vi "Switchmatrix Loop.vi"(6 "Used functions":bool, 8 "error in":errorcluster, 9 "IBM OptoElectroMechanics Configuration":T1={"Parameter Analizer"={"Parameter Analyzer VISA Session"="COM1", "Sweeping Time Parameters"={"Integration Time"=0, "Short Integration Time (s)"=1.0, "Long Integration Time (s)"=0.0, "Wait Time Parameter"=1.0}, "Acquisition Mode"=enum."Sweeping Mode", "Status Polling Time (ms)"=0, "Comment"="Test VI", "SMU 1 - Sweeping"={"Start / Offset"=0.0, "Stop / Ratio"=1.0, "Step \n(linear only)"=0.01, "Compliance"=0.1, "Power \nCompliance"=0.0, "Mode"=0, "Function"=0, "Sweep Mode"=FALSE}, "SMU 2 - Sweeping"={"Start / Offset"=0.0, "Stop / Ratio"=1.0, "Step \n(linear only)"=0.01, "Compliance"=0.1, "Power \nCompliance"=0.0, "Mode"=0, "Function"=0, "Sweep Mode"=FALSE}, "SMU 3 - Sweeping"={"Start / Offset"=0.0, "Stop / Ratio"=1.0, "Step \n(linear only)"=0.01, "Compliance"=0.1, "Power \nCompliance"=0.0, "Mode"=0, "Function"=0, "Sweep Mode"=FALSE}, "SMU 4 - Sweeping"={"Start / Offset"=0.0, "Stop / Ratio"=1.0, "Step \n(linear only)"=0.01, "Compliance"=0.1, "Power \nCompliance"=0.0, "Mode"=0, "Function"=0, "Sweep Mode"=FALSE}, "Sweep Spacing"=0, "Range"=0, "SMU1 - Sampling"={"Source"=10.0, "Compliance"=1e-05, "Mode"=0, "Function"=FALSE}, "SMU2 - Sampling"={"Source"=1.0, "Compliance"=1.0, "Mode"=0, "Function"=FALSE}, "SMU3 - Sampling"={"Source"=10.0, "Compliance"=1e-05, "Mode"=0, "Function"=FALSE}, "SMU4 - Sampling"={"Source"=0.1, "Compliance"=60.0, "Mode"=10, "Function"=FALSE}, "Sampling Time Parameters"={"Initial Interval (s)"=0.1, "Number of Samples"=60, "Total Sampling Time (s)"=10.0, "Hold Time (s)"=0.0, "Sampling Mode"=0, "Sampling Time"=0}, "Stop Condition"={"Enable Delay (s)"=0.0, "Name"="", "Threshold"=0.0, "num. of events"=1, "Event"=0, "Stop Condition Enable"=FALSE}}, "Switching Matrix"={"Switching Matrix VISA Session"="GPIB0::18::INSTR", "Connections"=[{"Connections"=[FALSE, FALSE, FALSE, FALSE, FALSE, FALSE, FALSE, FALSE, FALSE, FALSE, FALSE, FALSE], "Connection Type"=enum."Disconnected"}, {"Connections"=[FALSE, FALSE, FALSE, FALSE, FALSE, FALSE, FALSE, FALSE, FALSE, FALSE, FALSE, FALSE], "Connection Type"=enum."Disconnected"}, {"Connections"=[FALSE, FALSE, FALSE, FALSE, FALSE, FALSE, FALSE, FALSE, FALSE, FALSE, FALSE, FALSE], "Connection Type"=enum."Disconnected"}, {"Connections"=[FALSE, FALSE, FALSE, FALSE, FALSE, FALSE, FALSE, FALSE, FALSE, FALSE, FALSE, FALSE], "Connection Type"=enum."Disconnected"}, {"Connections"=[FALSE, FALSE, FALSE, FALSE, FALSE, FALSE, FALSE, FALSE, FALSE, FALSE, FALSE, FALSE], "Connection Type"=enum."Disconnected"}, {"Connections"=[FALSE, FALSE, FALSE, FALSE, FALSE, FALSE, FALSE, FALSE, FALSE, FALSE, FALSE, FALSE], "Connection Type"=enum."Disconnected"}, {"Connections"=[FALSE, FALSE, FALSE, FALSE, FALSE, FALSE, FALSE, FALSE, FALSE, FALSE, FALSE, FALSE], "Connection Type"=enum."Disconnected"}, {"Connections"=[FALSE, FALSE, FALSE, FALSE, FALSE, FALSE, FALSE, FALSE, FALSE, FALSE, FALSE, FALSE], "Connection Type"=enum."Disconnected"}]}, "Stress Control"={"Stress Control VISA Session"="StrainMotor", "Axis"=0, "Motion"=0, "Destination (°)"=0.0, "Speed (°/s)"=4.0, "Position (°)"=25.0}, "Optical Spectrometer"={"Laser Settings"={"Laser Wavelength"=enum."365 nm", "Neutral Density Filter"=enum."100%"}, "Spectrometer Settings"={"Confocal Hole Size (µm)"=0.0, "Grating"=2, "Detector"=enum."InGaAs Array"}, "Acquisition Settings"={"Acquisition Mode"=enum."Multi-Window", "Spectal Position (nm)"=632.0, "From (nm)"=735.0, "To (nm)"=0.0, "Integration Time (s)"=0.0, "Number of Accumulations"=3, "AutoScanning"=FALSE, "Spike Removal"=FALSE}, "Path"=path "C:/07 - Prizes and Awards/Marie Curie Prize/Reply Editors Final NCOMMS(10).docx"}, "Switches & Mirrors"={"Relay VISA Session"="COM1", "Switches"={"Laser"=FALSE, "Video"=FALSE}, "Delays (ms)"={"Laser"=500, "Video"=1500}}, "Camera"={"Settings"={"Pixel clock"=20, "Frame rate"=30.0, "Exposure time"=33.21525, "Master Gain"=0, "Red Gain"=0, "Green Gain"=0, "Blue Gain"=0, "Auto Gain"=FALSE, "White-balance"=FALSE, "Color Correction"=FALSE}}, "XYZ Stage"={"Connection Settings"={"Tango VISA"="", "Baudrate"=57600, "Show Protocol?"=FALSE}, "Manual Control"={"North"=FALSE, "South"=FALSE, "West"=FALSE, "East"=FALSE, "Up"=FALSE, "Down"=FALSE, "Stop"=FALSE, "XY Step"=0.0, "Z step"=0.0}, "Coordinate Control"={"Motion Mode"=enum."Absolute", "Destination [mm]"=[]}}, "AutoFocus"={"Matching Criteria"={"Minimum Score"=700.0, "Color Score Weight"=700.0, "Minimum Contrast"=50, "Match Mode"=0, "Match Feature Mode"=0, "Subpixel Accuracy"=TRUE, "Color Sensitivity"=1, "Search Strategy"=1}, "Z Scan Parameters"={"Z Range"=1380.0, "Resolution"=5000.0, "Initial Direction"=enum."Up", "Focus Threshold"=0.1, "Ascent Constant"=0.1}, "Displacement"=0.0, "Transformation Matrix"=[]}, "Sava Data"={"Workspace Info"={"Device Name"="ProberHead_Tst_C29K3_7(2)", "Device Info"="ProberHead_Tst_C29", "Path"=path "C:/Users/gio/Desktop/ProbeHeadTest"}, "Instrument Configuration"={"Instrument"=enum."Unknown Instrument", "Configuration"="Test Configuration"}, "Stress Motor Position"=0.0, "Electrical Measurement"={"Sequence"=[], "V1"=[], "V2"=[], "V3"=[], "V4"=[], "I1"=[], "I2"=[], "I3"=[], "I4"=[]}, "Optical Spectrum"={"Intensity"=[], "Wavelength"=[], "Energy"=[], "Raman Shift"=[], "Detector Temperature"=0.0}}, "PlotData"={"Sliders"={"Strain Sequence"=0, "Instrument Sequence"=0}, "Measurement"={"Which Instrument?"=enum."No Plot", "Electrical Measurement"={"Sequence"=[], "V1"=[], "V2"=[], "V3"=[], "V4"=[], "I1"=[], "I2"=[], "I3"=[], "I4"=[]}, "Measurement Mode"=enum."Sweeping Mode", "Optical Spectrum"={"Intensity"=[], "Wavelength"=[], "Energy"=[], "Raman Shift"=[], "Detector Temperature"=0.0}}, "Instrument Steps"=[], "Strain Points"=[]}, "Instrument Sequence"={"Caller VI"=enum."User"}, "Strain Measurement"={"Stress Sequence "={"Max Motor Position"=1380.0, "# Intermediate Points"=5000, "Initial Direction"=enum."Tension"}, "Track?"=FALSE}} {"AutoFocus"."Displacement" scale=1.0..1000.0; "AutoFocus"."Z Scan Parameters"."Focus Threshold" min=0.0 max=1000.0 step=1.0 format="%#_2f"; "AutoFocus"."Z Scan Parameters"."Ascent Constant" min=0.0 max=1000.0 step=1.0 format="%#_2f"; "AutoFocus"."Z Scan Parameters"."Resolution" min=0.0 max=1.0 step=0.01 format="%_2g"; "AutoFocus"."Z Scan Parameters"."Z Range" format="%_3g"; "AutoFocus"."Matching Criteria"."Match Mode" items=["Shift Invariant", "Rotation Invariant"]; "AutoFocus"."Matching Criteria"."Match Feature Mode" items=["Color and Shape", "Color", "Shape"]; "AutoFocus"."Matching Criteria"."Color Sensitivity" items=["Low Sensitivity", "Medium Sensitivity", "High Sensitivity"]; "AutoFocus"."Matching Criteria"."Search Strategy" items=["Conservative", "Balance", "Aggressive", "Very Aggressive"]; "XYZ Stage"."Manual Control"."Z step" scale=0.1..10.0; "XYZ Stage"."Manual Control"."XY Step" scale=0.1..1000.0; "Camera"."Settings"."Blue Gain" min=0 max=100 scale=0.0..100.0; "Camera"."Settings"."Green Gain" min=0 max=100 scale=0.0..100.0; "Camera"."Settings"."Red Gain" min=0 max=100 scale=0.0..100.0; "Camera"."Settings"."Master Gain" min=0 max=100 scale=0.0..100.0; "Camera"."Settings"."Exposure time" min=0.101625 max=159.246375 step=0.101625 scale=0.101625..159.246375 scale format="%#.3g"; "Camera"."Settings"."Frame rate" min=2.7455631699174137 max=6.2675785993528725 step=0.000101625 scale=2.7455631699174137..6.2675785993528725 scale format="%^#_3g"; "Camera"."Settings"."Pixel clock" min=5 max=43 scale=5.0..43.0; "PlotData"."Sliders"."Instrument Sequence" scale=0.0..10.0; "PlotData"."Sliders"."Strain Sequence" scale=0.0..10.0; "Strain Measurement"."Stress Sequence"."# Intermediate Points" max=1390; "Parameter Analizer"."Stop Condition"."Event" items=["Value > Threshold", "Value < Threshold", "| Value | > | Threshold |", "| Value | < | Threshold |"]; "Parameter Analizer"."Stop Condition"."Threshold" format="%^.2e"; "Parameter Analizer"."Stop Condition"."Enable Delay (s)" format="%.1f"; "Parameter Analizer"."Sampling Time Parameters"."Sampling Time" items=["Auto (linear only)", "No Limit", "Set Limit"]; "Parameter Analizer"."Sampling Time Parameters"."Sampling Mode" items=["Linear", "Log10", "Log25", "Log50", "Thinned Out"]; "Parameter Analizer"."Sampling Time Parameters"."Hold Time (s)" format="%.4f"; "Parameter Analizer"."Sampling Time Parameters"."Total Sampling Time (s)" format="%.1f"; "Parameter Analizer"."Sampling Time Parameters"."Initial Interval (s)" format="%^.3e"; "Parameter Analizer"."SMU 4 - Sweeping"."Function" items=["Disabled", "Var 1", "Var 2", "Var 1'", "Constant"]; "Parameter Analizer"."SMU 4 - Sweeping"."Mode" items=["V", "I", "V pulse", "I  pulse", "Common"]; "Parameter Analizer"."SMU 4 - Sweeping"."Power \nCompliance" format="%^.2e"; "Parameter Analizer"."SMU 4 - Sweeping"."Compliance" format="%^.2e"; "Parameter Analizer"."SMU 4 - Sweeping"."Step \n(linear only)" format="%^.4e"; "Parameter Analizer"."SMU 4 - Sweeping"."Stop / Ratio" format="%^.4e"; "Parameter Analizer"."SMU 4 - Sweeping"."Start / Offset" format="%^.4e"; "Parameter Analizer"."SMU 3 - Sweeping"."Function" items=["Disabled", "Var 1", "Var 2", "Var 1'", "Constant"]; "Parameter Analizer"."SMU 3 - Sweeping"."Mode" items=["V", "I", "V pulse", "I  pulse", "Common"]; "Parameter Analizer"."SMU 3 - Sweeping"."Power \nCompliance" format="%^.2e"; "Parameter Analizer"."SMU 3 - Sweeping"."Compliance" format="%^.2e"; "Parameter Analizer"."SMU 3 - Sweeping"."Step \n(linear only)" format="%^.4e"; "Parameter Analizer"."SMU 3 - Sweeping"."Stop / Ratio" format="%^.4e"; "Parameter Analizer"."SMU 3 - Sweeping"."Start / Offset" format="%^.4e"; "Parameter Analizer"."SMU 2 - Sweeping"."Function" items=["Disabled", "Var 1", "Var 2", "Var 1'", "Constant"]; "Parameter Analizer"."SMU 2 - Sweeping"."Mode" items=["V", "I", "V pulse", "I  pulse", "Common"]; "Parameter Analizer"."SMU 2 - Sweeping"."Power \nCompliance" format="%^.2e"; "Parameter Analizer"."SMU 2 - Sweeping"."Compliance" format="%^.2e"; "Parameter Analizer"."SMU 2 - Sweeping"."Step \n(linear only)" format="%^.4e"; "Parameter Analizer"."SMU 2 - Sweeping"."Stop / Ratio" format="%^.4e"; "Parameter Analizer"."SMU 2 - Sweeping"."Start / Offset" format="%^.4e"; "Parameter Analizer"."SMU 1 - Sweeping"."Function" items=["Disabled", "Var 1", "Var 2", "Var 1'", "Constant"]; "Parameter Analizer"."SMU 1 - Sweeping"."Mode" items=["V", "I", "V pulse", "I  pulse", "Common"]; "Parameter Analizer"."SMU 1 - Sweeping"."Power \nCompliance" format="%^.2e"; "Parameter Analizer"."SMU 1 - Sweeping"."Compliance" format="%^.2e"; "Parameter Analizer"."SMU 1 - Sweeping"."Step \n(linear only)" format="%^.4e"; "Parameter Analizer"."SMU 1 - Sweeping"."Stop / Ratio" format="%^.4e"; "Parameter Analizer"."SMU 1 - Sweeping"."Start / Offset" format="%^.4e"; "Parameter Analizer"."Sweeping Time Parameters"."Long Integration Time (s)" scale=0.02..2.0; "Parameter Analizer"."Sweeping Time Parameters"."Short Integration Time (s)" scale=8e-05..0.00192; "Parameter Analizer"."Sweeping Time Parameters"."Integration Time" items=["Short", "Long"]; "Parameter Analizer"."Sweeping Time Parameters"."Wait Time Parameter" format="%.1f"; "Parameter Analizer"."SMU4 - Sampling"."Mode" items=["V", "I", "Common"]; "Parameter Analizer"."SMU4 - Sampling"."Compliance" format="%^.2e"; "Parameter Analizer"."SMU4 - Sampling"."Source" format="%^.3e"; "Parameter Analizer"."SMU3 - Sampling"."Mode" items=["V", "I", "Common"]; "Parameter Analizer"."SMU3 - Sampling"."Compliance" format="%^.2e"; "Parameter Analizer"."SMU3 - Sampling"."Source" format="%^.3e"; "Parameter Analizer"."SMU2 - Sampling"."Mode" items=["V", "I", "Common"]; "Parameter Analizer"."SMU2 - Sampling"."Compliance" format="%^.2e"; "Parameter Analizer"."SMU2 - Sampling"."Source" format="%^.3e"; "Parameter Analizer"."SMU1 - Sampling"."Mode" items=["V", "I", "Common"]; "Parameter Analizer"."SMU1 - Sampling"."Compliance" format="%^.2e"; "Parameter Analizer"."SMU1 - Sampling"."Source" format="%^.3e"; "Parameter Analizer"."Range" items=["auto", "fixed", "limited"]; "Parameter Analizer"."Sweep Spacing" items=["linear", "log 10", "log 25", "log 50"]; "Stress Control"."Axis" min=1 max=3; "Stress Control"."Position (°)" format="%.6g"; "Stress Control"."Speed (°/s)" min=0.0 max=4.0 format="%.6f"; "Stress Control"."Destination (°)" min=-2000000000.0 max=2000000000.0 format="%.6f"; "Stress Control"."Motion" items=["Absolute", "Relative"]; "Optical Spectrometer"."Spectrometer Settings"."Grating" items=["1800 l/mm", "150 l/mm"]}, 10 "Message Queues out":T57, 11 "Notifiers":T44) -> (0 "error out":errorcluster)   [LabVIEW 2014]
uses:
  support/Message Queue/All Message Queues.ctl
  support/Message Queue/Message Cluster.ctl
  support/Notifiers/Notifiers.ctl
  support/Message Handler Loop Notifiers.ctl
  Hardware Control/Parameter Analyzer/Parameter Analyzer Notifiers.ctl
  Hardware Control/Switching Matrix/Switching Matrix Notifiers.ctl
  Hardware Control/Stress Control/StressControl Notifiers.ctl
  Hardware Control/Spectrometer/Spectrometer Notifiers.ctl
  Hardware Control/Switches and Mirrors/SwitchesMirrors Notifiers.ctl
  Hardware Control/Camera/Camera Notifiers.ctl
  Hardware Control/XYZ Stage/XYZ Notifications.ctl
  Hardware Control/Autofocus/Autofocus Notifiers.ctl
  Measurements/Optoelectronic Measurement/Optoelectronic Notifiers.ctl
  Measurements/Save Data/SaveData Notifiers.ctl
  Measurements/Instrument Sequence/Instrument Sequence Notifiers.ctl
  support/Configuration/Configuration.ctl
  Hardware Control/Parameter Analyzer/Parameter Analyzer Config.ctl
  Hardware Control/Parameter Analyzer/Parameter Analyzer Integration Parameters.ctl
  Hardware Control/Parameter Analyzer/Parameter Analyzer SMU Sweeping.ctl
  Hardware Control/Parameter Analyzer/Parameter Analyzer Sweep Spacing.ctl
  Hardware Control/Parameter Analyzer/Parameter Analyzer SMU Range.ctl
  Hardware Control/Parameter Analyzer/Parameter Analyzer SMU Sampling.ctl
  Hardware Control/Parameter Analyzer/Parameter Analyzer Sampling Parameters.ctl
  Hardware Control/Parameter Analyzer/Parameter Analyzer Stop Sampling Conditions.ctl
  Hardware Control/Switching Matrix/Switching Matrix Config.ctl
  Hardware Control/Stress Control/StressControl Config.ctl
  Hardware Control/Spectrometer/Spectrometer Config.ctl
  Hardware Control/Spectrometer/Laser Settings.ctl
  Hardware Control/Spectrometer/Laser.ctl
  Hardware Control/Spectrometer/Filter.ctl
  Hardware Control/Spectrometer/Grating Detector Settings.ctl
  Hardware Control/Spectrometer/Grating.ctl
  Hardware Control/Spectrometer/Detector.ctl
  Hardware Control/Spectrometer/Acquisition Settings.ctl
  Hardware Control/Switches and Mirrors/SwitchesMirrors Config.ctl
  Hardware Control/Switches and Mirrors/SwitchesMirrors Status.ctl
  Hardware Control/Camera/Camera Config.ctl
  Hardware Control/Camera/Camera Settings.ctl
  Hardware Control/XYZ Stage/XYZ Config.ctl
  Hardware Control/XYZ Stage/XYZ Connection Settings.ctl
  Hardware Control/XYZ Stage/XYZ Stage Control.ctl
  Hardware Control/XYZ Stage/XYZ Coordinate Control.ctl
  Hardware Control/Autofocus/AutoFocus Config.ctl
  Hardware Control/Autofocus/ZScan.ctl
  <vilib>/Analysis/Matrix/Datatypes/RealMatrix.ctl
  Measurements/Save Data/SaveData Config.ctl
  Measurements/Save Data/SaveData Workspace Info.ctl
  Measurements/Save Data/SaveData Instrument Configuration.ctl
  Measurements/Instrument Sequence/Instrument List.ctl
  Hardware Control/Spectrometer/Spectral Data.ctl
  Measurements/Plot Data/PlotData Config.ctl
  Measurements/Plot Data/Measurement.ctl
  Measurements/Plot Data/WhichInstrument.ctl
  Hardware Control/Parameter Analyzer/Electrical Data.ctl
  Measurements/Instrument Sequence/Instrument Steps.ctl
  Measurements/Instrument Sequence/Action.ctl
  Measurements/Instrument Sequence/Instrument Sequence Config.ctl
  Measurements/Strain Measurement/Strain Measurement Config.ctl
  support/Message Queue/Message Queue.lvlib
  <vilib>/Analysis/Matrix/NI_Matrix.lvlib
panel:
  # "LICENSED MATERIALS – PROPERTY OF IBM\nCopyright IBM Corp. 2016,\nALL RIGHTS RESERVED"
  # "XY"
  # "Z"
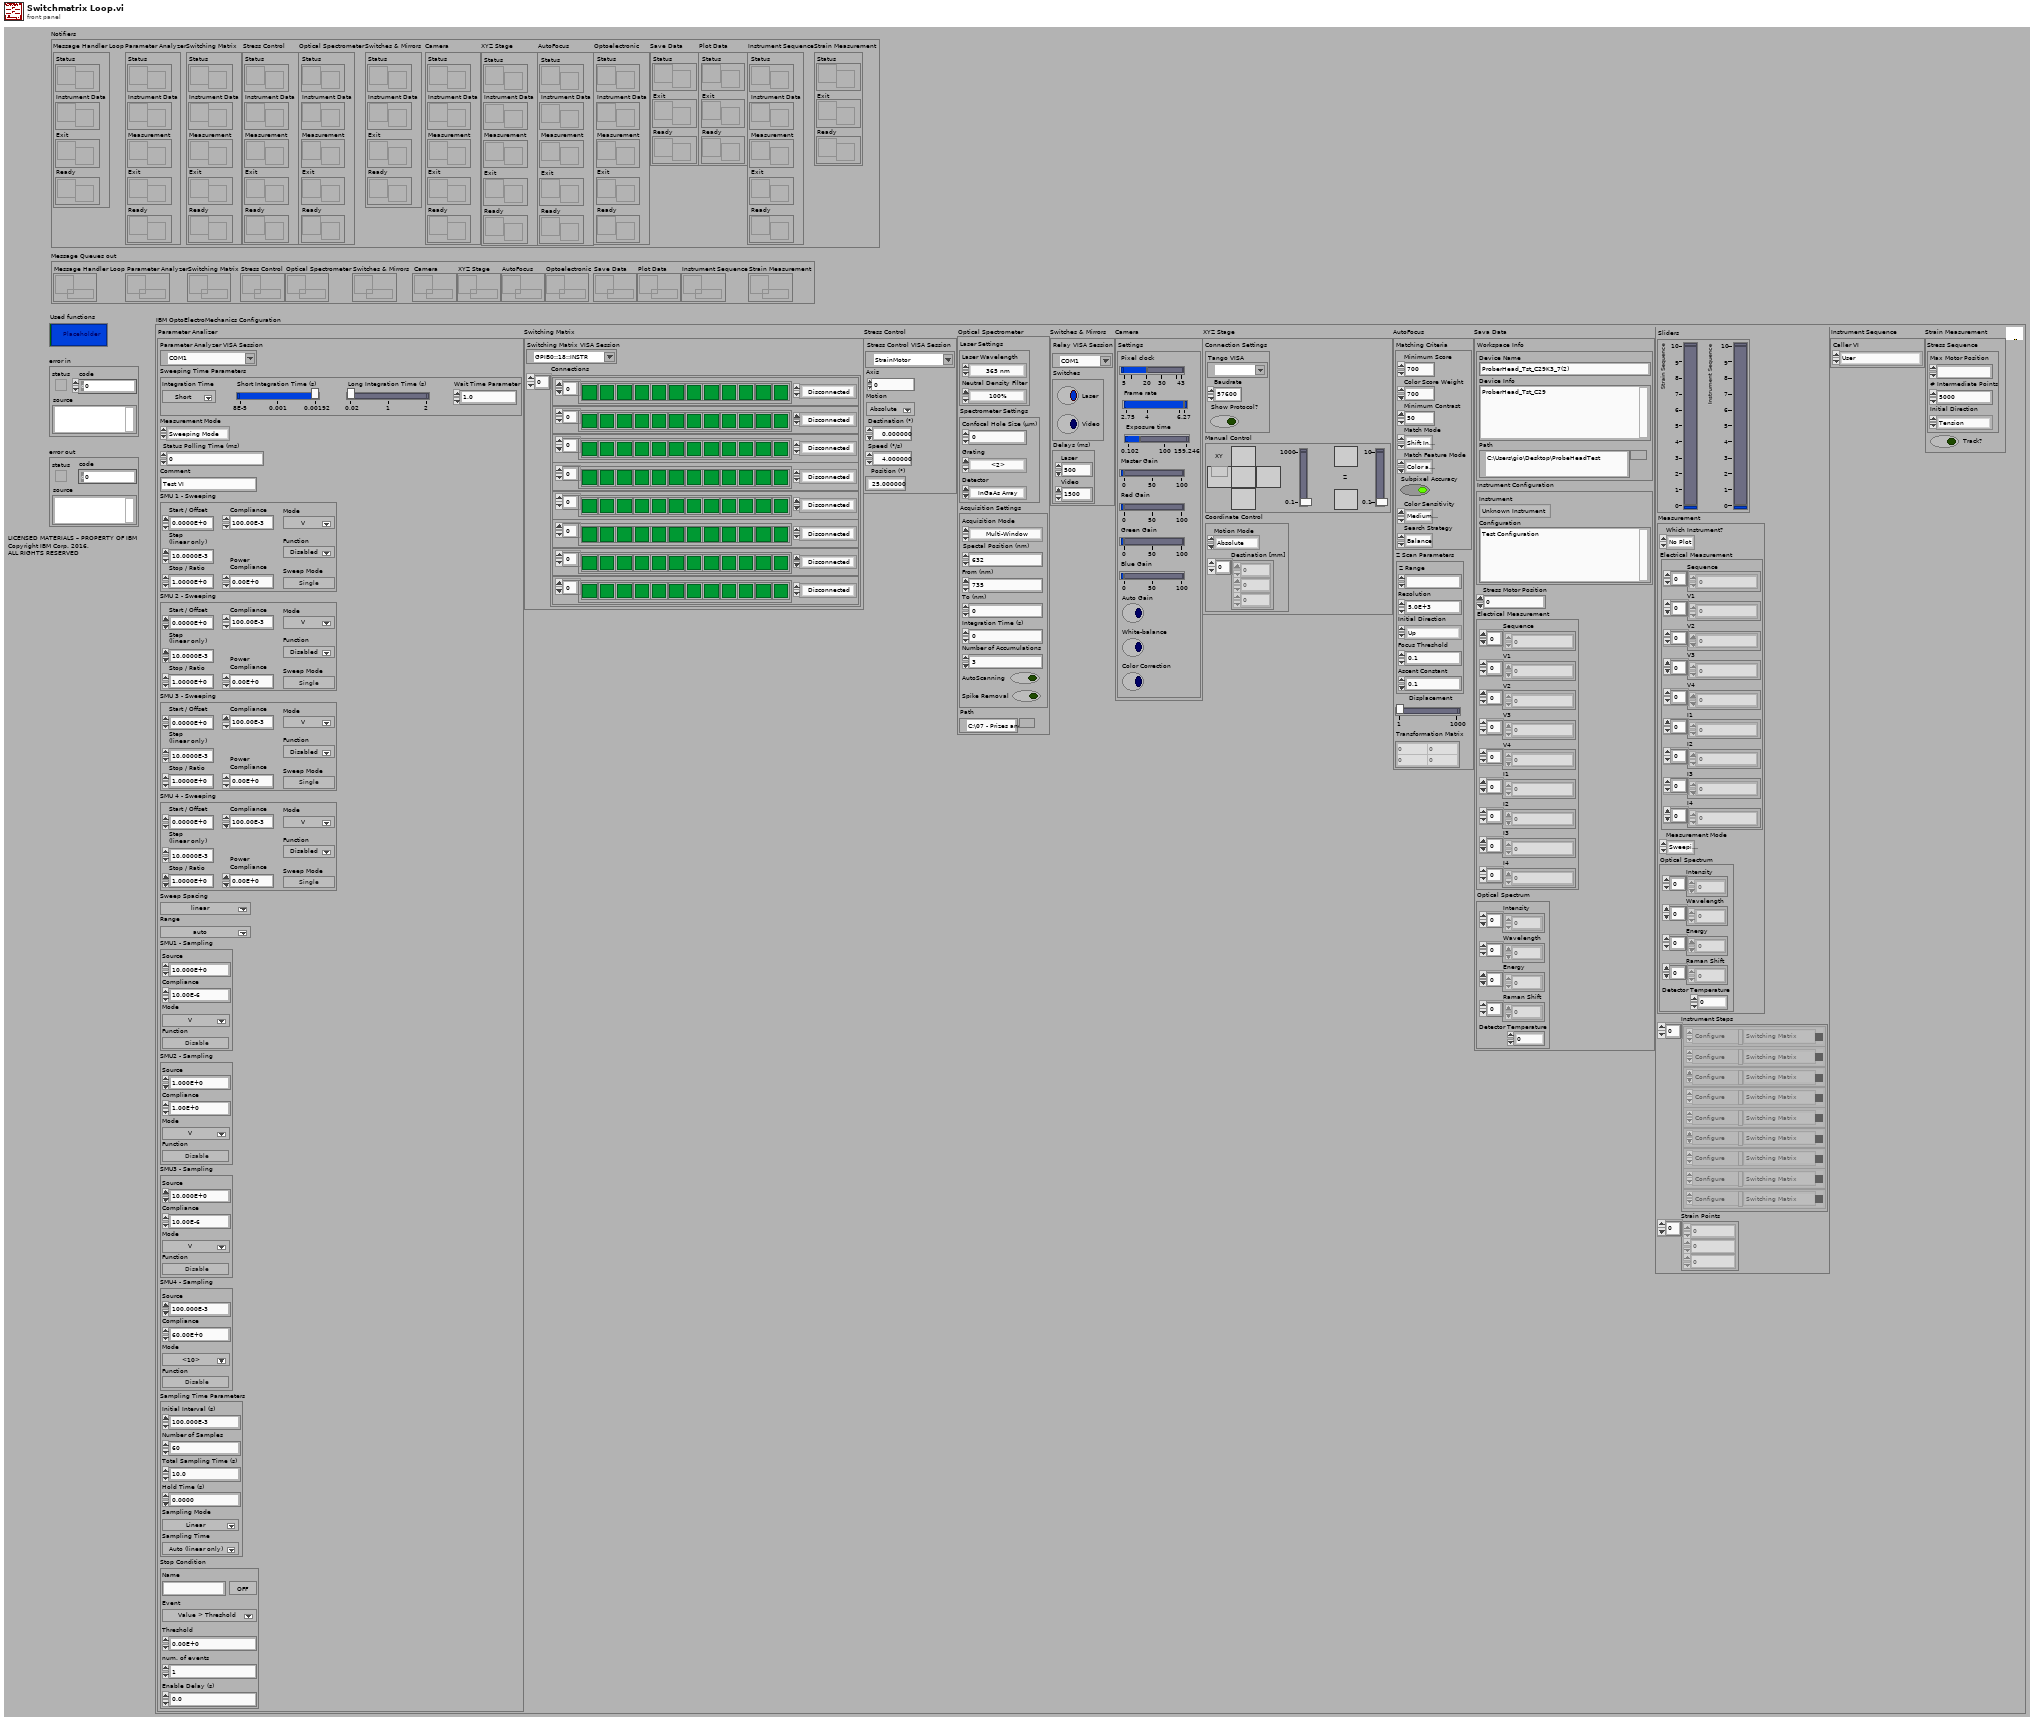
[diagram p1: front panel]
types:
  T1 = typedef "Configuration.ctl" = cluster{"Parameter Analizer":T2, "Switching Matrix":T10, "Stress Control":T11, "Optical Spectrometer":T12, "Switches & Mirrors":T20, "Camera":T22, "XYZ Stage":T24, "AutoFocus":T28, "Sava Data":T31, "PlotData":T36, "Instrument Sequence":T42, "Strain Measurement":T43}
  T2 = typedef "Parameter Analyzer Config.ctl" = cluster{"Parameter Analyzer VISA Session":refnum<visa-resource-name>, "Sweeping Time Parameters":T3, "Acquisition Mode":enum32{"Sweeping Mode", "Sampling Mode"}, "Status Polling Time (ms)":u32, "Comment":string, "SMU 1 - Sweeping":T4, "SMU 2 - Sweeping":T4, "SMU 3 - Sweeping":T4, "SMU 4 - Sweeping":T4, "Sweep Spacing":T5, "Range":T6, "SMU1 - Sampling":T7, "SMU2 - Sampling":T7, "SMU3 - Sampling":T7, "SMU4 - Sampling":T7, "Sampling Time Parameters":T8, "Stop Condition":T9}
  T3 = typedef "Parameter Analyzer Integration Parameters.ctl" = cluster{"Integration Time":u32, "Short Integration Time (s)":dbl, "Long Integration Time (s)":dbl, "Wait Time Parameter":dbl}
  T4 = typedef "Parameter Analyzer SMU Sweeping.ctl" = cluster{"Start / Offset":dbl, "Stop / Ratio":dbl, "Step \n(linear only)":dbl, "Compliance":dbl, "Power \nCompliance":dbl, "Mode":u32, "Function":i32, "Sweep Mode":bool}
  T5 = typedef "Parameter Analyzer Sweep Spacing.ctl" = u16
  T6 = typedef "Parameter Analyzer SMU Range.ctl" = u16
  T7 = typedef "Parameter Analyzer SMU Sampling.ctl" = cluster{"Source":dbl, "Compliance":dbl, "Mode":u32, "Function":bool}
  T8 = typedef "Parameter Analyzer Sampling Parameters.ctl" = cluster{"Initial Interval (s)":dbl, "Number of Samples":i32, "Total Sampling Time (s)":dbl, "Hold Time (s)":dbl, "Sampling Mode":i32, "Sampling Time":i32}
  T9 = typedef "Parameter Analyzer Stop Sampling Conditions.ctl" = cluster{"Enable Delay (s)":dbl, "Name":string, "Threshold":dbl, "num. of events":i32, "Event":i32, "Stop Condition Enable":bool}
  T10 = typedef "Switching Matrix Config.ctl" = cluster{"Switching Matrix VISA Session":refnum<visa-resource-name>, "Connections":cluster{"Connections":bool[], "Connection Type":enum16{"Disconnected", "Make - Break", "Break - Make"}}[]}
  T11 = typedef "StressControl Config.ctl" = cluster{"Stress Control VISA Session":refnum<visa-resource-name>, "Axis":i32, "Motion":u16, "Destination (°)":dbl, "Speed (°/s)":dbl, "Position (°)":dbl}
  T12 = typedef "Spectrometer Config.ctl" = cluster{"Laser Settings":T13, "Spectrometer Settings":T16, "Acquisition Settings":T19, "Path":path}
  T13 = typedef "Laser Settings.ctl" = cluster{"Laser Wavelength":T14, "Neutral Density Filter":T15}
  T14 = typedef "Laser.ctl" = enum16{"633 nm", "784 nm", "532 nm", "365 nm"}
  T15 = typedef "Filter.ctl" = enum16{"100%", "50%", "25%", "10%", "1%", "0.1%", "0.01%"}
  T16 = typedef "Grating Detector Settings.ctl" = cluster{"Confocal Hole Size (µm)":dbl, "Grating":T17, "Detector":T18}
  T17 = typedef "Grating.ctl" = u16
  T18 = typedef "Detector.ctl" = enum16{"InGaAs Array", "Silicon CCD"}
  T19 = typedef "Acquisition Settings.ctl" = cluster{"Acquisition Mode":enum16{"Single Window", "Multi-Window"}, "Spectal Position (nm)":dbl, "From (nm)":dbl, "To (nm)":dbl, "Integration Time (s)":dbl, "Number of Accumulations":i32, "AutoScanning":bool, "Spike Removal":bool}
  T20 = typedef "SwitchesMirrors Config.ctl" = cluster{"Relay VISA Session":refnum<visa-resource-name>, "Switches":T21, "Delays (ms)":cluster{"Laser":u32, "Video":u32}}
  T21 = typedef "SwitchesMirrors Status.ctl" = cluster{"Laser":bool, "Video":bool}
  T22 = typedef "Camera Config.ctl" = cluster{"Settings":T23}
  T23 = typedef "Camera Settings.ctl" = cluster{"Pixel clock":i32, "Frame rate":dbl, "Exposure time":dbl, "Master Gain":i32, "Red Gain":i32, "Green Gain":i32, "Blue Gain":i32, "Auto Gain":bool, "White-balance":bool, "Color Correction":bool}
  T24 = typedef "XYZ Config.ctl" = cluster{"Connection Settings":T25, "Manual Control":T26, "Coordinate Control":T27}
  T25 = typedef "XYZ Connection Settings.ctl" = cluster{"Tango VISA":refnum<visa-resource-name>, "Baudrate":i32, "Show Protocol?":bool}
  T26 = typedef "XYZ Stage Control.ctl" = cluster{"North":bool, "South":bool, "West":bool, "East":bool, "Up":bool, "Down":bool, "Stop":bool, "XY Step":dbl, "Z step":dbl}
  T27 = typedef "XYZ Coordinate Control.ctl" = cluster{"Motion Mode":enum16{"Absolute", "Relative"}, "Destination [mm]":dbl[]}
  T28 = typedef "AutoFocus Config.ctl" = cluster{"Matching Criteria":cluster{"Minimum Score":sgl, "Color Score Weight":sgl, "Minimum Contrast":i32, "Match Mode":u32, "Match Feature Mode":u32, "Subpixel Accuracy":bool, "Color Sensitivity":u32, "Search Strategy":u32}, "Z Scan Parameters":T29, "Displacement":dbl, "Transformation Matrix":T30}
  T29 = typedef "ZScan.ctl" = cluster{"Z Range":ext, "Resolution":dbl, "Initial Direction":enum16{"Up", "Down"}, "Focus Threshold":dbl, "Ascent Constant":dbl}
  T30 = typedef "NI_Matrix.lvlib/RealMatrix.ctl" = dbl[][]
  T31 = typedef "SaveData Config.ctl" = cluster{"Workspace Info":T32, "Instrument Configuration":T33, "Stress Motor Position":dbl, "Electrical Measurement":cluster{"Sequence":dbl[], "V1":dbl[], "V2":dbl[], "V3":dbl[], "V4":dbl[], "I1":dbl[], "I2":dbl[], "I3":dbl[], "I4":dbl[]}, "Optical Spectrum":T35}
  T32 = typedef "SaveData Workspace Info.ctl" = cluster{"Device Name":string, "Device Info":string, "Path":path}
  T33 = typedef "SaveData Instrument Configuration.ctl" = cluster{"Instrument":T34, "Configuration":string}
  T34 = typedef "Instrument List.ctl" = enum32{"Unknown Instrument", "Switching Matrix", "Parameter Analyzer", "Optical Spectrometer", "Optoelectronic", "Autofocus"}
  T35 = typedef "Spectral Data.ctl" = cluster{"Intensity":dbl[], "Wavelength":dbl[], "Energy":dbl[], "Raman Shift":dbl[], "Detector Temperature":dbl}
  T36 = typedef "PlotData Config.ctl" = cluster{"Sliders":cluster{"Strain Sequence":i32, "Instrument Sequence":i32}, "Measurement":T37, "Instrument Steps":T40, "Strain Points":dbl[]}
  T37 = typedef "Measurement.ctl" = cluster{"Which Instrument?":T38, "Electrical Measurement":T39, "Measurement Mode":enum16{"Sweeping Mode", "Sampling Mode"}, "Optical Spectrum":T35}
  T38 = typedef "WhichInstrument.ctl" = enum16{"No Plot", "Spectrometer", "Parameter Analyzer", "Optoelectronic"}
  T39 = typedef "Electrical Data.ctl" = cluster{"Sequence":dbl[], "V1":dbl[], "V2":dbl[], "V3":dbl[], "V4":dbl[], "I1":dbl[], "I2":dbl[], "I3":dbl[], "I4":dbl[]}
  T40 = typedef "Instrument Steps.ctl" = cluster{"Action":T41, "Configuration":variant, "Instrument":T34, "Status":enum8{"False", "True", "Mixed"}}[]
  T41 = typedef "Action.ctl" = enum32{"Configure", "Measure"}
  T42 = typedef "Instrument Sequence Config.ctl" = cluster{"Caller VI":enum16{"User", "Stress Measurement VI"}}
  T43 = typedef "Strain Measurement Config.ctl" = cluster{"Stress Sequence ":cluster{"Max Motor Position":ext, "# Intermediate Points":u32, "Initial Direction":enum16{"Tension", "Compression"}}, "Track?":bool}
  T44 = typedef "Notifiers.ctl" = cluster{"Message Handler Loop":T45, "Parameter Analyzer":T46, "Switching Matrix":T47, "Stress Control":T48, "Optical Spectrometer":T49, "Switches & Mirrors":T50, "Camera":T51, "XYZ Stage":T52, "AutoFocus":T53, "Optoelectronic":T54, "Save Data":T55, "Plot Data":T55, "Instrument Sequence":T56, "Strain Measurement":cluster{"Status":refnum<notifier>, "Exit":refnum<notifier>, "Ready":refnum<notifier>}}
  T45 = typedef "Message Handler Loop Notifiers.ctl" = cluster{"Status":refnum<notifier>, "Instrument Data":refnum<notifier>, "Exit":refnum<notifier>, "Ready":refnum<notifier>}
  T46 = typedef "Parameter Analyzer Notifiers.ctl" = cluster{"Status":refnum<notifier>, "Instrument Data":refnum<notifier>, "Measurement":refnum<notifier>, "Exit":refnum<notifier>, "Ready":refnum<notifier>}
  T47 = typedef "Switching Matrix Notifiers.ctl" = cluster{"Status":refnum<notifier>, "Instrument Data":refnum<notifier>, "Measurement":refnum<notifier>, "Exit":refnum<notifier>, "Ready":refnum<notifier>}
  T48 = typedef "StressControl Notifiers.ctl" = cluster{"Status":refnum<notifier>, "Instrument Data":refnum<notifier>, "Measurement":refnum<notifier>, "Exit":refnum<notifier>, "Ready":refnum<notifier>}
  T49 = typedef "Spectrometer Notifiers.ctl" = cluster{"Status":refnum<notifier>, "Instrument Data":refnum<notifier>, "Measurement":refnum<notifier>, "Exit":refnum<notifier>, "Ready":refnum<notifier>}
  T50 = typedef "SwitchesMirrors Notifiers.ctl" = cluster{"Status":refnum<notifier>, "Instrument Data":refnum<notifier>, "Exit":refnum<notifier>, "Ready":refnum<notifier>}
  T51 = typedef "Camera Notifiers.ctl" = cluster{"Status":refnum<notifier>, "Instrument Data":refnum<notifier>, "Measurement":refnum<notifier>, "Exit":refnum<notifier>, "Ready":refnum<notifier>}
  T52 = typedef "XYZ Notifications.ctl" = cluster{"Status":refnum<notifier>, "Instrument Data":refnum<notifier>, "Measurement":refnum<notifier>, "Exit":refnum<notifier>, "Ready":refnum<notifier>}
  T53 = typedef "Autofocus Notifiers.ctl" = cluster{"Status":refnum<notifier>, "Instrument Data":refnum<notifier>, "Measurement":refnum<notifier>, "Exit":refnum<notifier>, "Ready":refnum<notifier>}
  T54 = typedef "Optoelectronic Notifiers.ctl" = cluster{"Status":refnum<notifier>, "Instrument Data":refnum<notifier>, "Measurement":refnum<notifier>, "Exit":refnum<notifier>, "Ready":refnum<notifier>}
  T55 = typedef "SaveData Notifiers.ctl" = cluster{"Status":refnum<notifier>, "Exit":refnum<notifier>, "Ready":refnum<notifier>}
  T56 = typedef "Instrument Sequence Notifiers.ctl" = cluster{"Status":refnum<notifier>, "Instrument Data":refnum<notifier>, "Measurement":refnum<notifier>, "Exit":refnum<notifier>, "Ready":refnum<notifier>}
  T57 = typedef "Message Queue.lvlib/All Message Queues.ctl" = cluster{"Message Handler Loop":refnum<queue>, "Parameter Analyzer":refnum<queue>, "Switching Matrix":refnum<queue>, "Stress Control":refnum<queue>, "Optical Spectrometer":refnum<queue>, "Switches & Mirrors":refnum<queue>, "Camera":refnum<queue>, "XYZ Stage":refnum<queue>, "AutoFocus":refnum<queue>, "Optoelectronic":refnum<queue>, "Save Data":refnum<queue>, "Plot Data":refnum<queue>, "Instrument Sequence":refnum<queue>, "Strain Measurement":refnum<queue>}
  T58 = typedef "Switching Matrix Data.ctl" = cluster{"Configuration":T10, "Refnums":T59, "Initialization":T60}
  T59 = typedef "Switching Matrix Refnums.ctl" = cluster{"Connections":refnum<vi>, "Instrument Status":refnum<vi>}
  T60 = typedef "Switching Matrix Initialization.ctl" = cluster{"Update Visa Session":bool, "Update Refnums":bool}
  T61 = enum32{"Connect", "Set Connections", "Get Connections", "Status Query", "Disconnect", "Update Refnums"}
  T62 = cluster{"Connections":bool[], "Connection Type":enum16{"Disconnected", "Make - Break", "Break - Make"}}[]
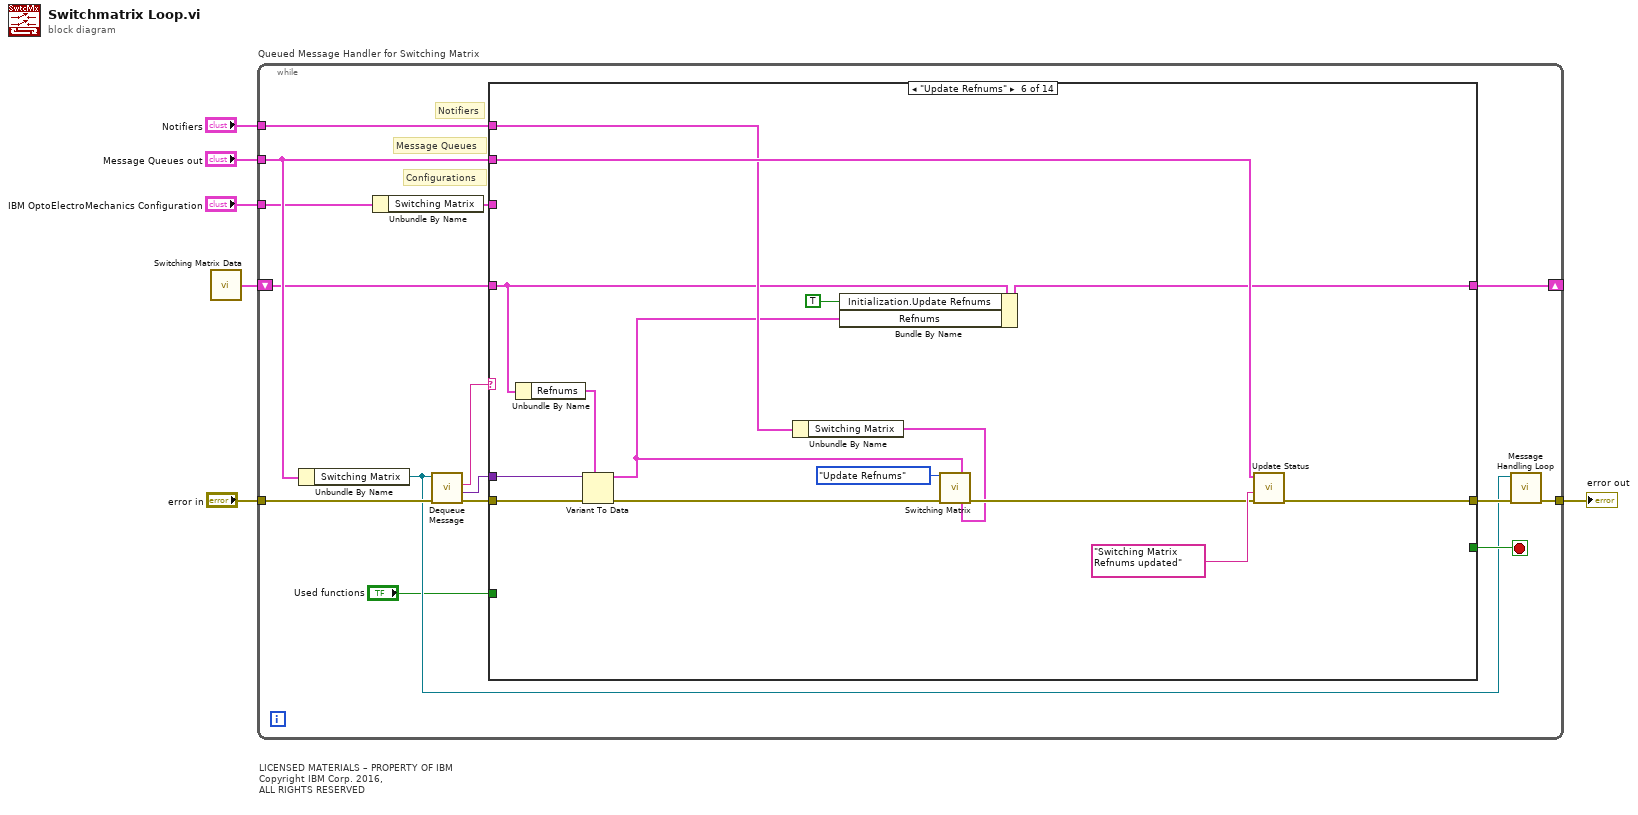
[diagram p0: block diagram]
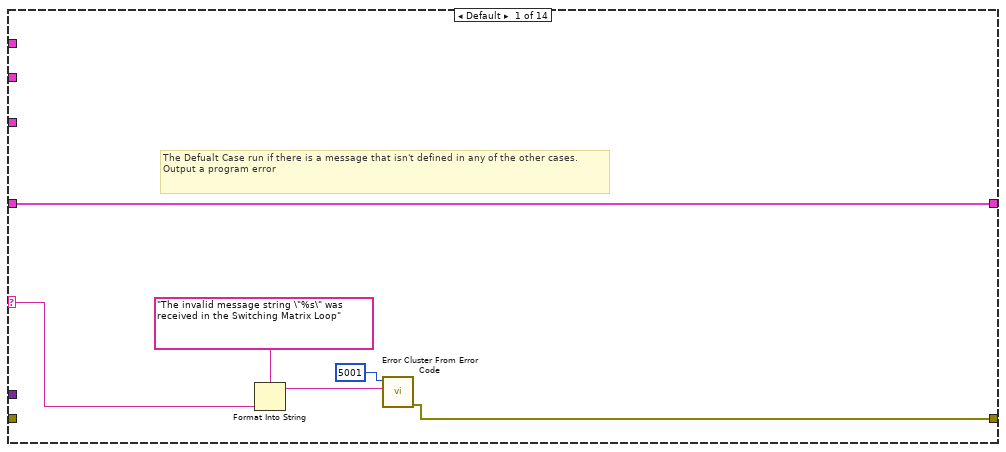
[diagram p2: hidden frame]
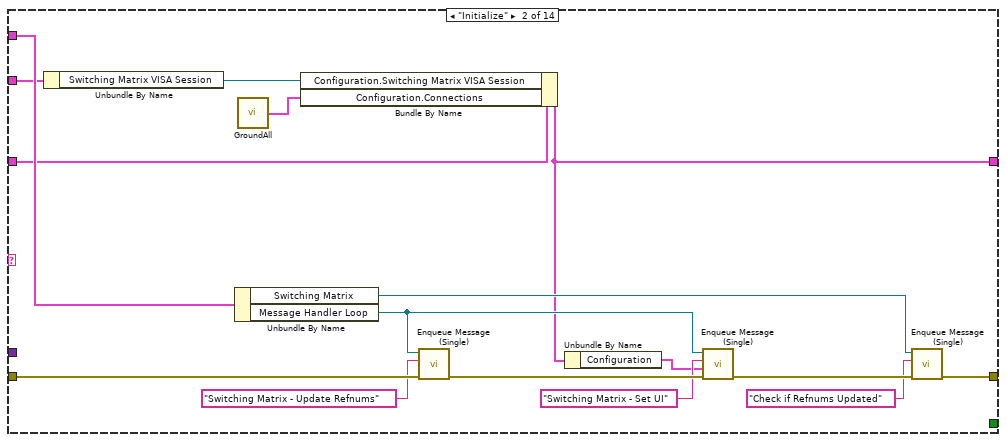
[diagram p3: hidden frame]
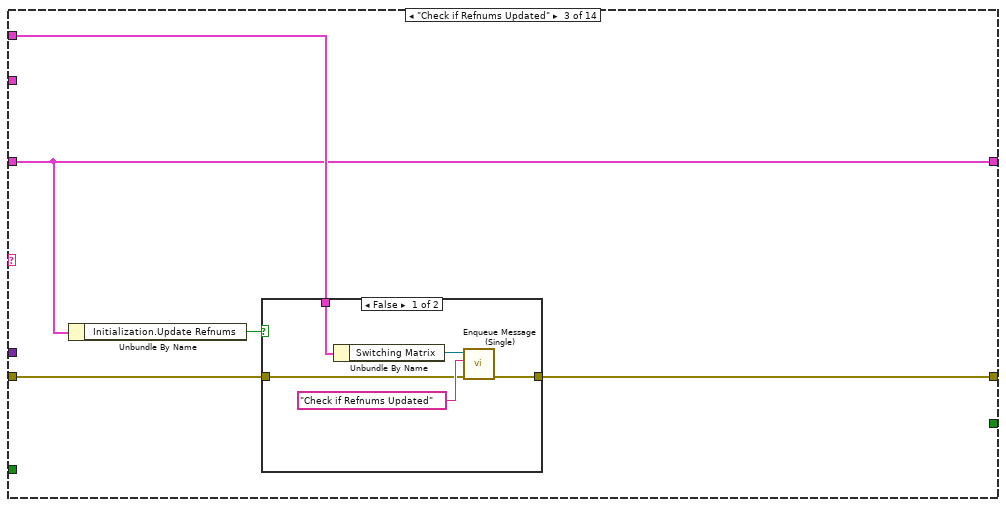
[diagram p4: hidden frame]
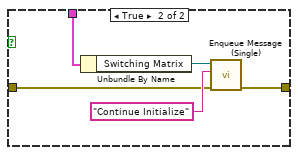
[diagram p5: hidden frame]
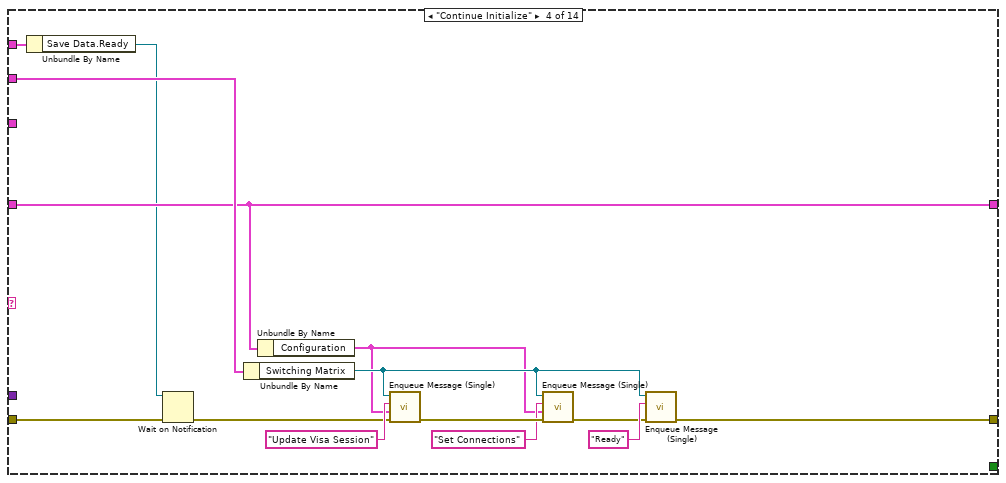
[diagram p6: hidden frame]
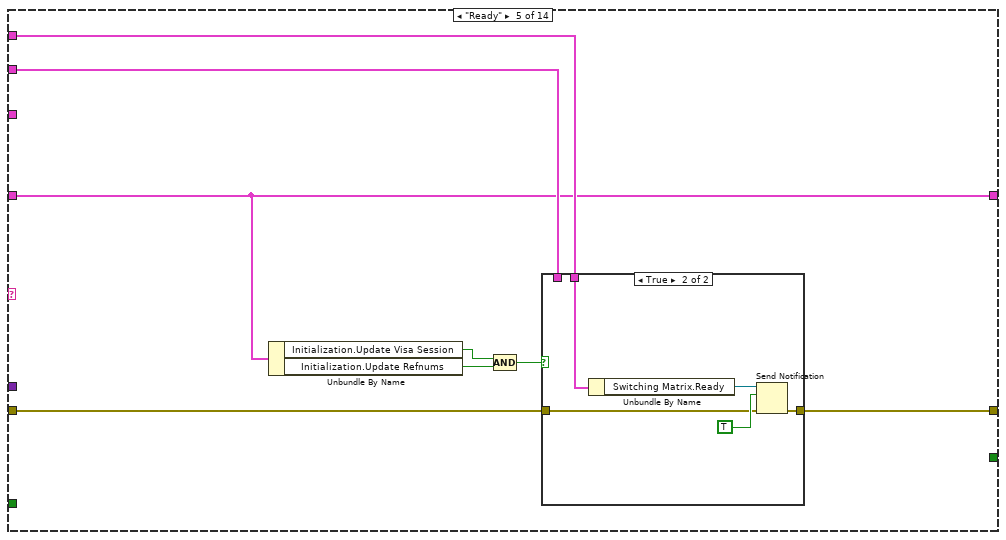
[diagram p7: hidden frame]
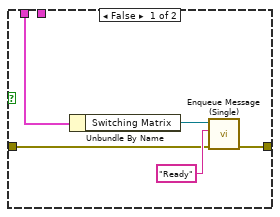
[diagram p8: hidden frame]
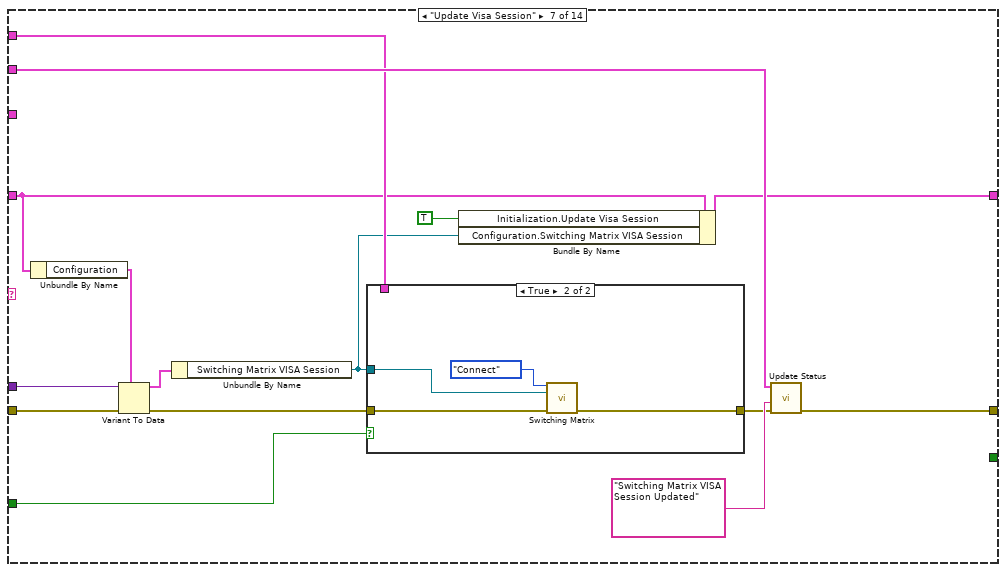
[diagram p9: hidden frame]
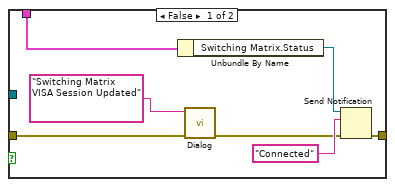
[diagram p10: hidden frame]
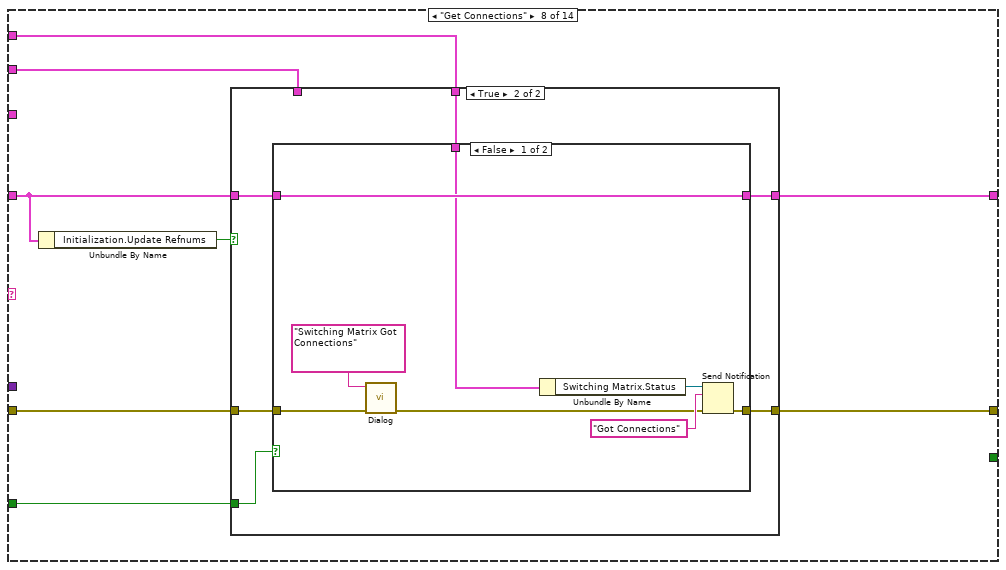
[diagram p11: hidden frame]
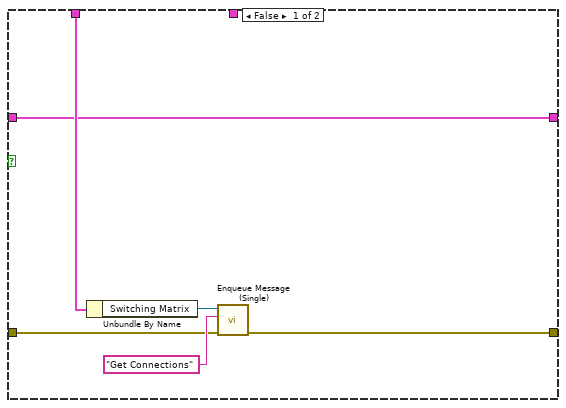
[diagram p12: hidden frame]
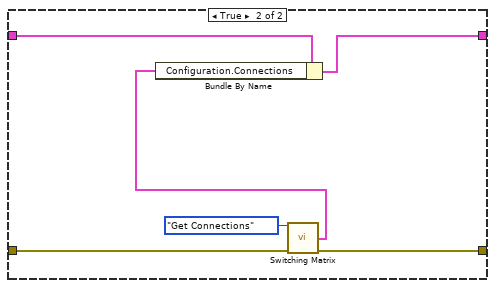
[diagram p13: hidden frame]
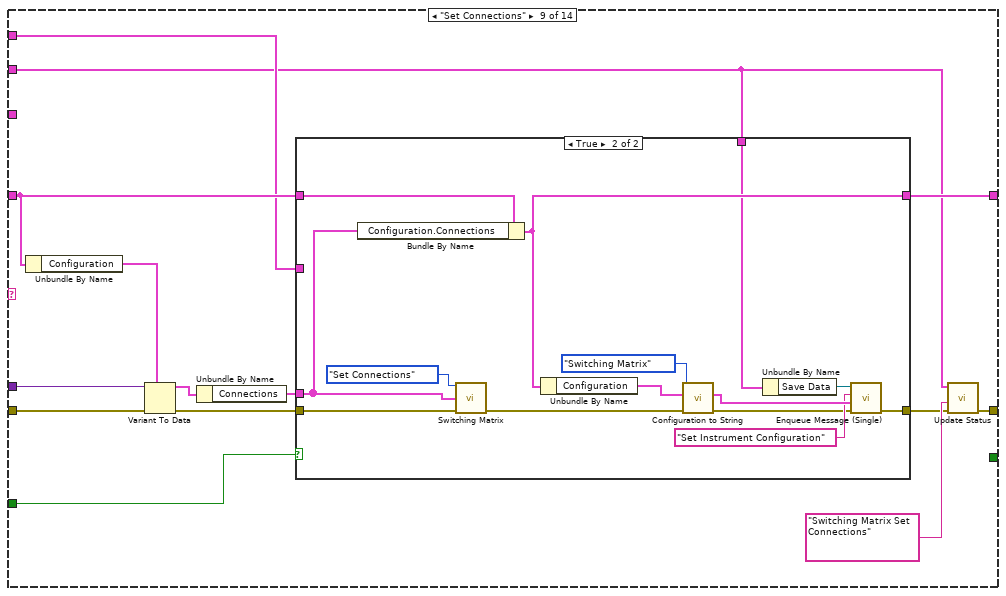
[diagram p14: hidden frame]
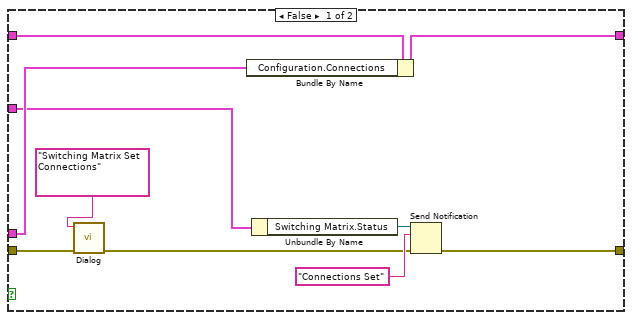
[diagram p15: hidden frame]
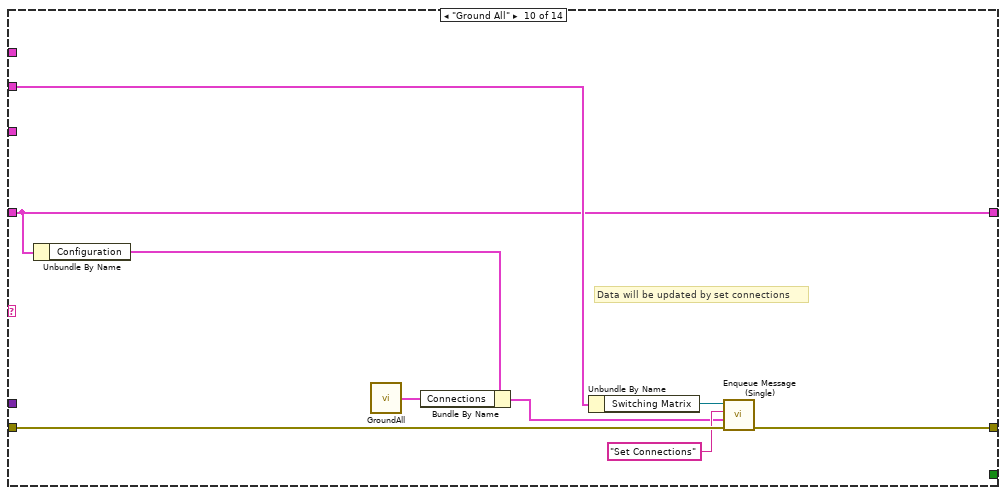
[diagram p16: hidden frame]
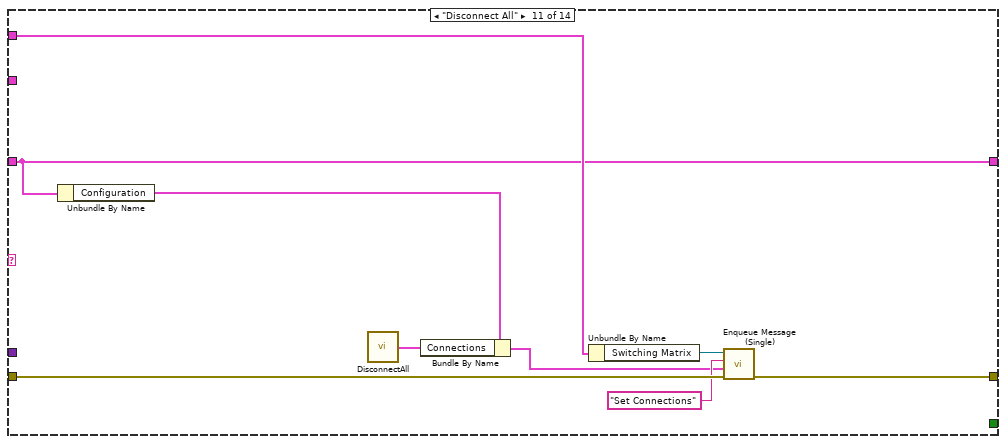
[diagram p17: hidden frame]
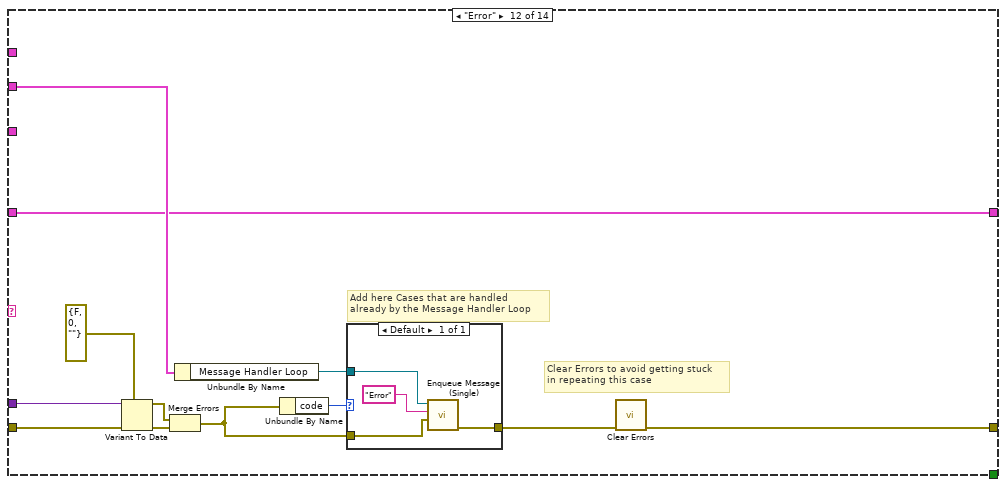
[diagram p18: hidden frame]
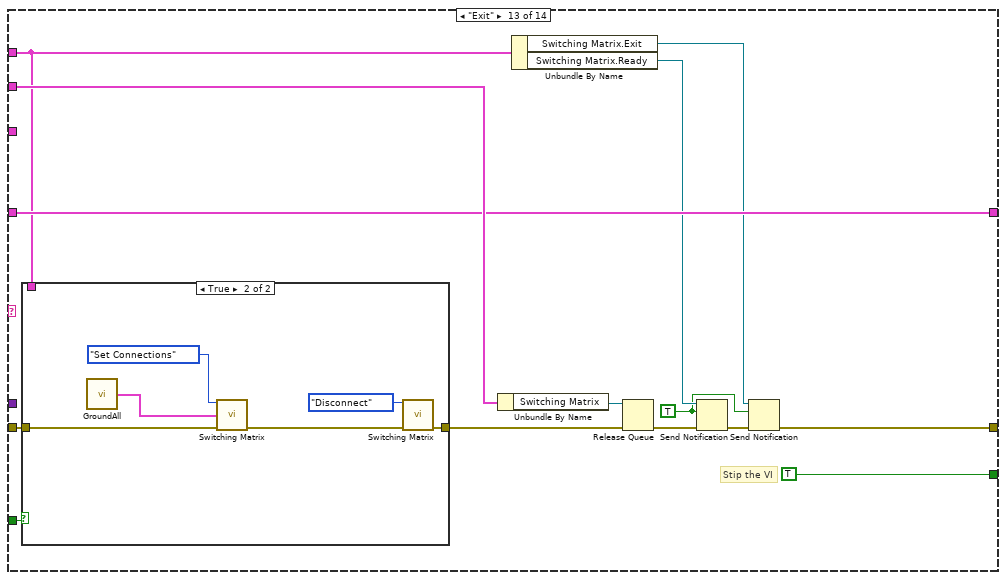
[diagram p19: hidden frame]
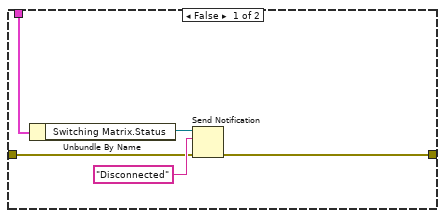
[diagram p20: hidden frame]
diagram:
  # "LICENSED MATERIALS – PROPERTY OF IBM\nCopyright IBM Corp. 2016,\nALL RIGHTS RESERVED"
  n1 = call "Switching Matrix Data.vi"() -> ("Keithley 707A Swithing Matrix Data"=w1:T58)
  n2 = while "Queued Message Handler for Switching Matrix" {
    tunnel: "error in" -> [w21]
    tunnel: [w13] -> w2
    tunnel: "Message Queues out" -> [w17]
    tunnel: "Notifiers" -> [w16]
    tunnel: "IBM OptoElectroMechanics Configuration" -> [w11]
    shift-right: [w7] -> _
    shift-left: w1 -> [w8]
    stop <- w15 stop-if-true
    # "Configurations"
    # "Notifiers"
    # "Message Queues"
    n3 = Unbundle By Name(w17) -> ("Switching Matrix"=w12:refnum<queue>)
    n4 = Unbundle By Name(w11) -> ("Switching Matrix"=w10:T10)
    n5 = call "Dequeue Message.vi"("error in (no error)"=w21, "Message Queue"=w12) -> ("error out"=w20:errorcluster, "Message Data"=w18:variant, "Message"=w19:string)  [unwired: 7 out]
    n6 = case shown="\"Update Refnums\"" w19 {
      selector: w19 -> [w24 _ _ _ _ _ _ _ _ _ _ _ _ _]
      tunnel: w20 -> [_ w41 w47 w60 w79 w104 w118 w139 w179 w210 w219 w230 w248 w267]
      tunnel: [w23 w32 w46 w71 w77 w103 w116 w133 w173 w207 w216 w225 w239 w266] -> w14
      tunnel: w18 -> [_ _ _ _ _ w105 w120 _ w176 _ _ w223 _ _]
      tunnel: w17 -> [_ w43 w48 w72 w78 w101 w115 w138 w166 w212 w221 w231 w250 _]
      tunnel: w16 -> [_ _ _ w61 w76 w100 w111 w132 w167 _ _ _ w238 w265]
      tunnel: [_ _ _ _ _ _ _ _ _ _ _ _ TRUE ("Priority Message? (F)") _] -> w15
      tunnel: w10 -> [_ w36 _ _ _ _ _ _ _ _ _ _ _ _]
      tunnel: w8 -> [w22 w42 w45 w64 w75 w93 w107 w137 w172 w205 w214 w222 w245 w263]
      tunnel: "Used functions" -> [_ _ _ _ _ _ w117 w134 w175 _ _ _ w246 _]
      tunnel: [w22 w29 w45 w64 w75 w99 w110 w135 w178 w205 w214 w222 w245 w263] -> w7
      frame Default {
        # "The Defualt Case run if there is a message that isn't defined in any of the other cases.\nOutput a program error"
        n7 = Format Into String(format string="The invalid message string \"%s\" was  received in the Switching Matrix Loop", w24) -> (resulting string=w26:string)  [unwired: 2 in, 1 out]
        n8 = call <vilib>:"Error Cluster From Error Code.vi"("error message (\"\")"=w26, "error code (0)"=5001) -> ("error out"=w23:errorcluster)  [unwired: 2 in, 5 out]
      }
      frame "Initialize" {
        n9 = Unbundle By Name(w36) -> ("Switching Matrix VISA Session"=w31:refnum<visa-resource-name>)
        n10 = Unbundle By Name(w43) -> ("Switching Matrix"=w34:refnum<queue>, "Message Handler Loop"=w38:refnum<queue>)
        n11 = call "GroundAll.vi"() -> ("Connections"=w30:T62)
        n12 = Bundle By Name(cluster=w42, "Configuration.Switching Matrix VISA Session"=w31, "Configuration.Connections"=w30) -> (w29:T58)
        n13 = call "Enqueue Message (Single).vi"("error in (no error)"=w41, "Message"="Switching Matrix - Update Refnums", "Message Queue"=w38) -> ("error out"=w39:errorcluster)  [unwired: 1 in, 7 out]
        n14 = Unbundle By Name(w29) -> ("Configuration"=w28:T10)
        n15 = call "Enqueue Message (Single).vi"("error in (no error)"=w39, "Message Data"=w28, "Message"="Switching Matrix - Set UI", "Message Queue"=w38) -> ("error out"=w35:errorcluster)  [unwired: 7 out]
        n16 = call "Enqueue Message (Single).vi"("error in (no error)"=w35, "Message"="Check if Refnums Updated", "Message Queue"=w34) -> ("error out"=w32:errorcluster)  [unwired: 1 in, 7 out]
      }
      frame "Check if Refnums Updated" {
        n17 = Unbundle By Name(w45) -> ("Initialization.Update Refnums"=w44:bool)
        n18 = case shown="False" w44 {
          tunnel: w48 -> [w53 w58]
          tunnel: w47 -> [w50 w55]
          tunnel: [w49 w54] -> w46
          frame False {
            n19 = Unbundle By Name(w53) -> ("Switching Matrix"=w52:refnum<queue>)
            n20 = call "Enqueue Message (Single).vi"("error in (no error)"=w50, "Message"="Check if Refnums Updated", "Message Queue"=w52) -> ("error out"=w49:errorcluster)  [unwired: 1 in, 7 out]
          }
          frame True {
            n21 = Unbundle By Name(w58) -> ("Switching Matrix"=w57:refnum<queue>)
            n22 = call "Enqueue Message (Single).vi"("error in (no error)"=w55, "Message"="Continue Initialize", "Message Queue"=w57) -> ("error out"=w54:errorcluster)  [unwired: 1 in, 7 out]
          }
        }
      }
      frame "Continue Initialize" {
        n23 = Unbundle By Name(w61) -> ("Save Data.Ready"=w62:refnum<notifier>)
        n24 = Wait on Notification(notifier=w62, error in (no error)=w60) -> (error out=w59:errorcluster)  [unwired: 2 in, 3 out]
        n25 = Unbundle By Name(w72) -> ("Switching Matrix"=w66:refnum<queue>)
        n26 = Unbundle By Name(w64) -> ("Configuration"=w63:T10)
        n27 = call "Enqueue Message (Single).vi"("error in (no error)"=w59, "Message Data"=w63, "Message"="Update Visa Session", "Message Queue"=w66) -> ("error out"=w69:errorcluster)  [unwired: 7 out]
        n28 = call "Enqueue Message (Single).vi"("error in (no error)"=w69, "Message Data"=w63, "Message"="Set Connections", "Message Queue"=w66) -> ("error out"=w68:errorcluster)  [unwired: 7 out]
        n29 = call "Enqueue Message (Single).vi"("error in (no error)"=w68, "Message"="Ready", "Message Queue"=w66) -> ("error out"=w71:errorcluster)  [unwired: 1 in, 7 out]
      }
      frame "Ready" {
        n30 = Unbundle By Name(w75) -> ("Initialization.Update Visa Session"=w74:bool, "Initialization.Update Refnums"=w73:bool)
        n31 = Compound Arithmetic op=AND(w74, w73) -> (w80:bool)
        n32 = case shown="True" w80 {
          tunnel: [w83 w88] -> w77
          tunnel: w79 -> [w82 w87]
          tunnel: w78 -> [w81 _]
          tunnel: w76 -> [_ w86]
          frame False {
            n33 = Unbundle By Name(w81) -> ("Switching Matrix"=w85:refnum<queue>)
            n34 = call "Enqueue Message (Single).vi"("error in (no error)"=w82, "Message"="Ready", "Message Queue"=w85) -> ("error out"=w83:errorcluster)  [unwired: 1 in, 7 out]
          }
          frame True {
            n35 = Unbundle By Name(w86) -> ("Switching Matrix.Ready"=w89:refnum<notifier>)
            n36 = Send Notification(notification=TRUE, notifier=w89, error in (no error)=w87) -> (error out=w88:errorcluster)  [unwired: 1 out]
          }
        }
      }
      frame "Update Refnums" {
        n37 = Unbundle By Name(w93) -> ("Refnums"=w92:T59)
        n38 = Variant To Data(error in=w104, type=w92, Variant=w105) -> (data=w91:T59, error out=w96:errorcluster)
        n39 = Unbundle By Name(w100) -> ("Switching Matrix"=w95:T47)
        n40 = Bundle By Name(cluster=w93, "Initialization.Update Refnums"=TRUE, "Refnums"=w91) -> (w99:T58)
        n41 = call "Switching Matrix.vi"("Function"=T61."Update Refnums", "SwitchMatrix Refnums"=w91, "error in"=w96, "Switchmatrix Notifications"=w95) -> ("error out"=w97:errorcluster)  [unwired: 6 in, 5 out]
        n42 = call "Update Status.vi"("error in"=w97, "String"="Switching Matrix Refnums updated" ("button name (\"OK\")"), "Message Queues out"=w101) -> ("error out"=w103:errorcluster)  [unwired: 8 out]
      }
      frame "Update Visa Session" {
        n43 = Unbundle By Name(w107) -> ("Configuration"=w106:T10)
        n44 = Variant To Data(error in=w118, type=w106, Variant=w120) -> (data=w113:T10, error out=w119:errorcluster)
        n45 = Unbundle By Name(w113) -> ("Switching Matrix VISA Session"=w108:refnum<visa-resource-name>)
        n46 = case shown="True" w117 {
          tunnel: w119 -> [w122 w131]
          tunnel: [w125 w130] -> w112
          tunnel: w108 -> [_ w129]
          tunnel: w111 -> [w127 _]
          frame False {
            n47 = Unbundle By Name(w127) -> ("Switching Matrix.Status"=w126:refnum<notifier>)
            n48 = call "Dialog.vi"("error in (no error)"=w122, "message"="Switching Matrix  VISA Session Updated" ("button name (\"OK\")")) -> ("error out"=w121:errorcluster)  [unwired: 1 in, 8 out]
            n49 = Send Notification(notification="Connected", notifier=w126, error in (no error)=w121) -> (error out=w125:errorcluster)  [unwired: 1 out]
          }
          frame True {
            n50 = call "Switching Matrix.vi"("Function"=T61."Connect", "VISA Resource Name"=w129, "error in"=w131) -> ("error out"=w130:errorcluster)  [unwired: 7 in, 5 out]
          }
        }
        n51 = Bundle By Name(cluster=w107, "Initialization.Update Visa Session"=TRUE, "Configuration.Switching Matrix VISA Session"=w108) -> (w110:T58)
        n52 = call "Update Status.vi"("error in"=w112, "String"="Switching Matrix VISA Session Updated" ("button name (\"OK\")"), "Message Queues out"=w115) -> ("error out"=w116:errorcluster)  [unwired: 8 out]
      }
      frame "Get Connections" {
        n53 = Unbundle By Name(w137) -> ("Initialization.Update Refnums"=w136:bool)
        n54 = case shown="True" w136 {
          tunnel: w139 -> [w143 w151]
          tunnel: w138 -> [w141 _]
          tunnel: w137 -> [w140 w150]
          tunnel: [w140 w149] -> w135
          tunnel: w134 -> [_ w148]
          tunnel: [w142 w147] -> w133
          tunnel: w132 -> [_ w146]
          frame False {
            n55 = Unbundle By Name(w141) -> ("Switching Matrix"=w144:refnum<queue>)
            n56 = call "Enqueue Message (Single).vi"("error in (no error)"=w143, "Message"="Get Connections", "Message Queue"=w144) -> ("error out"=w142:errorcluster)  [unwired: 1 in, 7 out]
          }
          frame True {
            n57 = case shown="False" w148 {
              tunnel: w151 -> [w158 w165]
              tunnel: [w153 w164] -> w147
              tunnel: w150 -> [w159 w162]
              tunnel: [w159 w161] -> w149
              tunnel: w146 -> [w152 _]
              frame False {
                n58 = call "Dialog.vi"("error in (no error)"=w158, "message"="Switching Matrix Got Connections" ("button name (\"OK\")")) -> ("error out"=w154:errorcluster)  [unwired: 1 in, 8 out]
                n59 = Unbundle By Name(w152) -> ("Switching Matrix.Status"=w155:refnum<notifier>)
                n60 = Send Notification(notification="Got Connections", notifier=w155, error in (no error)=w154) -> (error out=w153:errorcluster)  [unwired: 1 out]
              }
              frame True {
                n61 = call "Switching Matrix.vi"("Function"=T61."Get Connections", "error in"=w165) -> ("Get Switch Matrix"=w160:T62, "error out"=w164:errorcluster)  [unwired: 8 in, 4 out]
                n62 = Bundle By Name(cluster=w162, "Configuration.Connections"=w160) -> (w161:T58)
              }
            }
          }
        }
      }
      frame "Set Connections" {
        n63 = Unbundle By Name(w172) -> ("Configuration"=w171:T10)
        n64 = Variant To Data(error in=w179, type=w171, Variant=w176) -> (data=w170:T10, error out=w177:errorcluster)
        n65 = Unbundle By Name(w170) -> ("Connections"=w169:T62)
        n66 = case shown="True" w175 {
          tunnel: [w181 w195] -> w168
          tunnel: [w188 w194] -> w178
          tunnel: w177 -> [w186 w203]
          tunnel: w172 -> [w189 w202]
          tunnel: w169 -> [w187 w200]
          tunnel: w167 -> [w180 _]
          tunnel: w166 -> [_ w193]
          frame False {
            n67 = call "Dialog.vi"("error in (no error)"=w186, "message"="Switching Matrix Set Connections" ("button name (\"OK\")")) -> ("error out"=w182:errorcluster)  [unwired: 1 in, 8 out]
            n68 = Bundle By Name(cluster=w189, "Configuration.Connections"=w187) -> (w188:T58)
            n69 = Unbundle By Name(w180) -> ("Switching Matrix.Status"=w184:refnum<notifier>)
            n70 = Send Notification(notification="Connections Set", notifier=w184, error in (no error)=w182) -> (error out=w181:errorcluster)  [unwired: 1 out]
          }
          frame True {
            n71 = Bundle By Name(cluster=w202, "Configuration.Connections"=w200) -> (w194:T58)
            n72 = call "Switching Matrix.vi"("Function"=T61."Set Connections", "Set Switch Matrix"=w200, "error in"=w203) -> ("error out"=w196:errorcluster)  [unwired: 7 in, 5 out]
            n73 = Unbundle By Name(w194) -> ("Configuration"=w191:T10)
            n74 = call "Configuration to String.vi"("error in (no error)"=w196, "Configuration"=w191, "Instrument"=Instrument_List."Switching Matrix") -> ("error out"=w197:errorcluster, "Instrument Configuration"=w199:T33)  [unwired: 7 out]
            n75 = Unbundle By Name(w193) -> ("Save Data"=w192:refnum<queue>)
            n76 = call "Enqueue Message (Single).vi"("error in (no error)"=w197, "Message Data"=w199, "Message"="Set Instrument Configuration", "Message Queue"=w192) -> ("error out"=w195:errorcluster)  [unwired: 7 out]
          }
        }
        n77 = call "Update Status.vi"("error in"=w168, "String"="Switching Matrix Set Connections" ("button name (\"OK\")"), "Message Queues out"=w166) -> ("error out"=w173:errorcluster)  [unwired: 8 out]
      }
      frame "Ground All" {
        # "Data will be updated by set connections"
        n78 = Unbundle By Name(w205) -> ("Configuration"=w209:T10)
        n79 = call "GroundAll.vi"() -> ("Connections"=w204:T62)
        n80 = Bundle By Name(cluster=w209, "Connections"=w204) -> (w206:T10)
        n81 = Unbundle By Name(w212) -> ("Switching Matrix"=w211:refnum<queue>)
        n82 = call "Enqueue Message (Single).vi"("error in (no error)"=w210, "Message Data"=w206, "Message"="Set Connections", "Message Queue"=w211) -> ("error out"=w207:errorcluster)  [unwired: 7 out]
      }
      frame "Disconnect All" {
        n83 = Unbundle By Name(w214) -> ("Configuration"=w218:T10)
        n84 = call "DisconnectAll.vi"() -> ("Connections"=w213:T62)
        n85 = Bundle By Name(cluster=w218, "Connections"=w213) -> (w215:T10)
        n86 = Unbundle By Name(w221) -> ("Switching Matrix"=w220:refnum<queue>)
        n87 = call "Enqueue Message (Single).vi"("error in (no error)"=w219, "Message Data"=w215, "Message"="Set Connections", "Message Queue"=w220) -> ("error out"=w216:errorcluster)  [unwired: 7 out]
      }
      frame "Error" {
        # "Clear Errors to avoid getting stuck \nin repeating this case"
        # "Add here Cases that are handled \nalready by the Message Handler Loop"
        n88 = Variant To Data(error in=w230, type=errorcluster {"status"=FALSE, "code"=0, "source"=""} ("error out"), Variant=w223) -> (data=w229:errorcluster, error out=w228:errorcluster)
        n89 = Merge Errors(w229, w228) -> (w227:errorcluster)
        n90 = Unbundle By Name(w231) -> ("Message Handler Loop"=w233:refnum<queue>)
        n91 = Unbundle By Name(w227) -> ("code"=w224:i32)
        n92 = case shown="Default" w224 {
          tunnel: w233 -> [w237]
          tunnel: w227 -> [w235]
          tunnel: [w234] -> w226
          frame Default {
            n93 = call "Enqueue Message (Single).vi"("Message Data"=w235, "Message"="Error", "Message Queue"=w237) -> ("error out"=w234:errorcluster)  [unwired: 1 in, 7 out]
          }
        }
        n94 = call <vilib>:"Clear Errors.vi"("error in (no error)"=w226) -> ("error out"=w225:errorcluster)  [unwired: 1 in, 5 out]
      }
      frame "Exit" {
        w242 = TRUE ("Priority Message? (F)")
        # "Stip the VI"
        n95 = case shown="True" w246 {
          tunnel: w248 -> [w254 w258]
          tunnel: [w253 w262] -> w247
          tunnel: w238 -> [w252 _]
          frame False {
            n96 = Unbundle By Name(w252) -> ("Switching Matrix.Status"=w255:refnum<notifier>)
            n97 = Send Notification(notification="Disconnected", notifier=w255, error in (no error)=w254) -> (error out=w253:errorcluster)  [unwired: 1 out]
          }
          frame True {
            n98 = call "GroundAll.vi"() -> ("Connections"=w257:T62)
            n99 = call "Switching Matrix.vi"("Function"=T61."Set Connections", "Set Switch Matrix"=w257, "error in"=w258) -> ("error out"=w259:errorcluster)  [unwired: 7 in, 5 out]
            n100 = call "Switching Matrix.vi"("Function"=T61."Disconnect", "error in"=w259) -> ("error out"=w262:errorcluster)  [unwired: 8 in, 5 out]
          }
        }
        n101 = Unbundle By Name(w250) -> ("Switching Matrix"=w251:refnum<queue>)
        n102 = Unbundle By Name(w238) -> ("Switching Matrix.Exit"=w241:refnum<notifier>, "Switching Matrix.Ready"=w244:refnum<notifier>)
        n103 = Release Queue(queue=w251, error in (no error)=w247) -> (error out=w240:errorcluster)  [unwired: 3 out]
        n104 = Send Notification(notification=w242, notifier=w244, error in (no error)=w240) -> (error out=w243:errorcluster)  [unwired: 1 out]
        n105 = Send Notification(notification=w242, notifier=w241, error in (no error)=w243) -> (error out=w239:errorcluster)  [unwired: 1 out]
      }
      frame "Notify Status" {
        n106 = Unbundle By Name(w265) -> ("Switching Matrix.Instrument Data"=w264:refnum<notifier>)
        n107 = Send Notification(notification=w263, notifier=w264, error in (no error)=w267) -> (error out=w266:errorcluster)  [unwired: 1 out]
      }
    }
    n108 = call "Message Handling Loop.vi"("error in (no error)"=w14, "Message Queue"=w12) -> ("dup error in"=w13:errorcluster)  [unwired: 9 out]
  }
  "error out" <- w2
